vi "Example6-Abstraction.vi"   [LabVIEW 2021]
doc: "Example of object abstraction in LabVIEW. Comments in Polish."
uses:
  Droid/Droid.lvclass
  BattleDroid/BattleDroid.lvclass
  Astromech droid/Astromech droid.lvclass
  MedicalDroid/MedicalDroid.lvclass
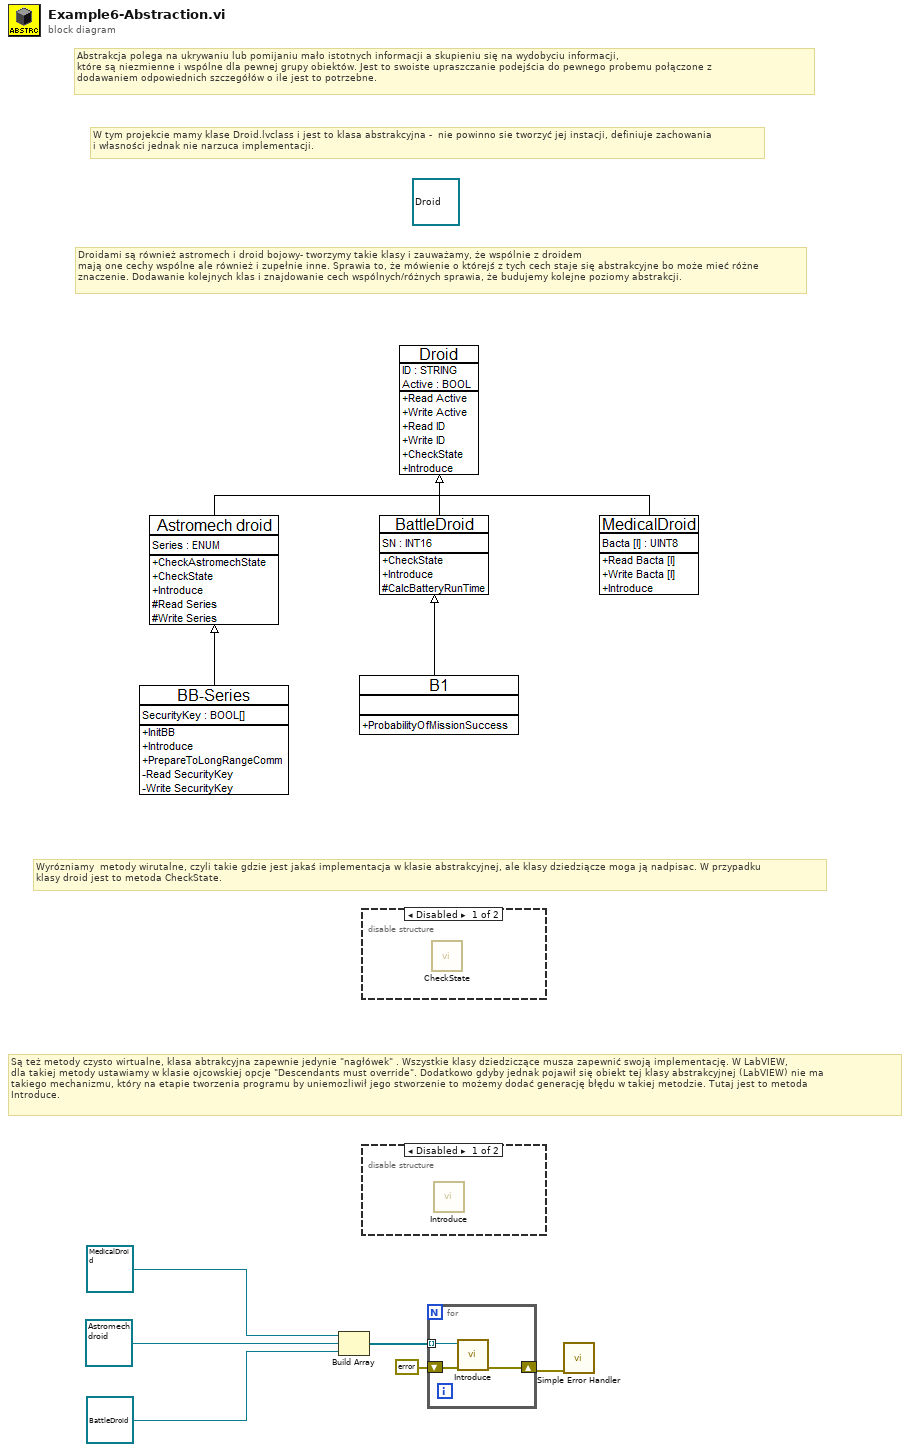
[diagram p0: block diagram]
diagram:
  (unwired) refnum<class "Droid.lvclass"> refnum ("Droid.lvclass")
  # "Są też metody czysto wirtualne, klasa abtrakcyjna zapewnie jedynie \"nagłówek\" . Wszystkie klasy dziedziczące musza zapewnić swoją implementację. W LabVIEW,\ndla takiej metody ustawiamy w klasie ojcowskiej opcje \"Descendants must override\". Dodatkowo gdyby jednak pojawił się obiekt tej klasy abstrakcyjnej (LabVIEW) nie ma \ntakiego mechanizmu, który na etapie tworzenia programu by uniemozliwił jego stworzenie to możemy dodać generację błędu w takiej metodzie. Tutaj jest to metoda \nIntroduce."
  # "Wyrózniamy  metody wirutalne, czyli takie gdzie jest jakaś implementacja w klasie abstrakcyjnej, ale klasy dziedziącze moga ją nadpisac. W przypadku\nklasy droid jest to metoda CheckState."
  # "Droidami są również astromech i droid bojowy- tworzymy takie klasy i zauważamy, że wspólnie z droidem\nmają one cechy wspólne ale również i zupełnie inne. Sprawia to, że mówienie o którejś z tych cech staje się abstrakcyjne bo może mieć różne \nznaczenie. Dodawanie kolejnych klas i znajdowanie cech wspólnych/różnych sprawia, że budujemy kolejne poziomy abstrakcji."
  # "W tym projekcie mamy klase Droid.lvclass i jest to klasa abstrakcyjna -  nie powinno sie tworzyć jej instacji, definiuje zachowania\ni własności jednak nie narzuca implementacji."
  # "Abstrakcja polega na ukrywaniu lub pomijaniu mało istotnych informacji a skupieniu się na wydobyciu informacji, \nktóre są niezmienne i wspólne dla pewnej grupy obiektów. Jest to swoiste upraszczanie podejścia do pewnego probemu połączone z \ndodawaniem odpowiednich szczegółów o ile jest to potrzebne."
  n1 = Build Array(refnum<class "MedicalDroid.lvclass"> refnum ("MedicalDroid.lvclass"), refnum<class "Astromech droid.lvclass"> refnum ("Astromech droid.lvclass"), refnum<class "BattleDroid.lvclass"> refnum ("BattleDroid.lvclass")) -> (w3:refnum<class "Droid.lvclass">[])
  n2 = disable-structure shown="Disabled" {
    frame Disabled {
      n3 = call-dynamic "CheckState.vi"() -> ()  [unwired: 10 in, 2 out]
    }
    frame Enabled {
    }
  }
  n4 = disable-structure shown="Disabled" {
    frame Disabled {
      n5 = call-dynamic "Introduce.vi"() -> ()  [unwired: 10 in, 2 out]
    }
    frame Enabled {
    }
  }
  n6 = for {
    tunnel: w3 -> [w9] mode=indexing
    shift-right: [w8] -> w2
    shift-left: errorcluster {"status"=FALSE, "code"=0, "source"=""} ("Error Out") -> [w7]
    n7 = call-dynamic "Introduce.vi"("Error In"=w7, "Droid in"=w9) -> ("Error Out"=w8:errorcluster)  [unwired: 8 in, 1 out]
  }
  n8 = call <vilib>:"Simple Error Handler.vi"("error in (no error)"=w2) -> ()  [unwired: 4 in, 5 out]
